vi "Get Header Ref.vi"(8 "error in (no error)":errorcluster, 11 "xwpfHeader in":refnum<class "xwpfHeader_Footer.lvclass">) -> (0 "error out":errorcluster, 2 "Header Ref":refnum<k24>, 3 "xwpfHeader out":refnum<class "xwpfHeader_Footer.lvclass">)   [LabVIEW 2017, in "Word_Specific.lvlib" / "xwpfHeader_Footer.lvclass"]
uses:
  xwpfHeader_Footer.lvclass
  C:/Users/Neo/Desktop/Dev_Tools_BR/LabVIEW_NPOI/src/lib/NPOI 2.1.1/NPOI.OOXML.dll
  lib/NPOI 2.1.1/NPOI.OOXML.dll
  xwpfHeader_Footer.lvclass/xwpfHeader_Footer.ctl
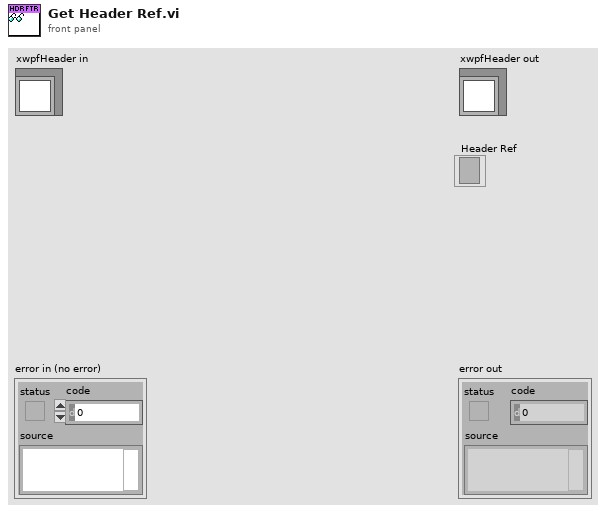
[diagram p1: front panel]
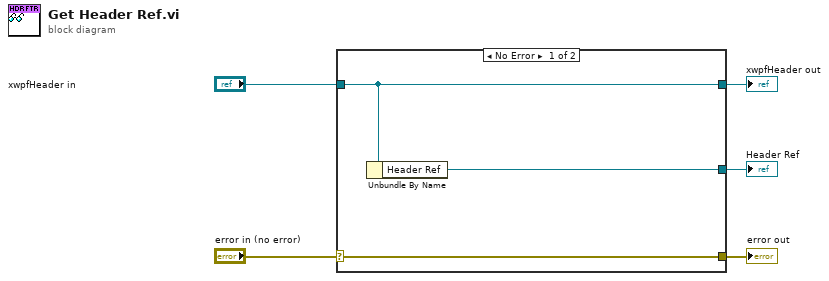
[diagram p0: block diagram]
diagram:
  n1 = case shown="No Error" "error in (no error)" {
    selector: "error in (no error)" -> [w8 w9]
    tunnel: [w8 w9] -> w4
    tunnel: [w7 w10] -> w2
    tunnel: "xwpfHeader in" -> [w7 w10]
    tunnel: [w6 _] -> w1
    frame No Error {
      n2 = Unbundle By Name(w7) -> ("Header Ref"=w6:refnum<k24>)
    }
    frame Error {
    }
  }
  "error out" <- w4
  "xwpfHeader out" <- w2
  "Header Ref" <- w1
